vi "Read Alias.vi"(11 "Attributes in":refnum<class "Attributes.lvclass">) -> (2 "Alias":string)   [LabVIEW 2020, in "jettl.lvlib" / "Attributes.lvclass"]
uses:
  Attributes.lvclass
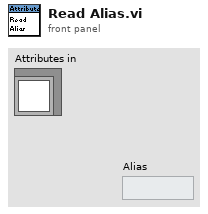
[diagram p1: front panel]
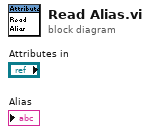
[diagram p0: block diagram]
diagram:
